vi "LS_DAQ_Cluster_RealTime.vi"() -> ()   [LabVIEW 2020]
uses:
  <vilib>/Platform/TimedLoop/XDataNode/timing_clust.ctl
  <vilib>/Platform/TimedLoop/XDataNode/nitl_modes.ctl
  <vilib>/Platform/TimedLoop/XDataNode/wakeup.ctl
  <vilib>/platform/TimedLoop/XDataNode/XDataNode.xnode
  <vilib>/Platform/TimedLoop/XDataNode/XDNodeRunTimeDep.lvlib
panel:
  out "Pulse count":dbl
  out "Period [ms]":u32
  out "Data":dbl[](array[numeric])
  out "error IO":errorcluster
  out "Finished Late? [i-1]":bool
  out "Iteration Duration":i64
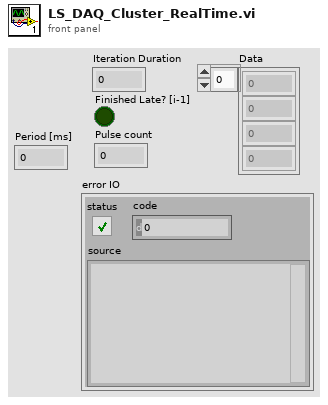
[diagram p1: front panel]
types:
  T1 = typedef "XDNodeRunTimeDep.lvlib/timing_clust.ctl" = cluster{"Expected End [f-1]":u64, "Actual End [f-1]":u64, "Finished Late? [f-1]":bool, "Expected End [i-1]":u64, "Actual End [i-1]":u64, "Finished Late? [i-1]":bool, "Expected Start [i]":u64, "Actual Start [i]":u64, "Expected Start [f]":u64, "Actual Start [f]":u64, "Source Name":string, "Structure Name":string, "Period":i64, "Deadline":i64, "Offset":i64, "Start":i64, "Priority":i32, "Timeout":i32, "Mode":T2, "Wakeup Reason":T3, "Error":errorcluster, "Source Type":string, "Secondary Source Type":string, "Global End Time":u64, "Global Start Time":u64, "Frame Duration":u64, "Iteration Duration":u64, "Assigned CPU":i32, "I/O Scan Engine Mode":u32}
  T2 = typedef "XDNodeRunTimeDep.lvlib/nitl_modes.ctl" = enum32{"No Change", "Process missed periods, maintain original phase", "Discard missed periods, maintain original phase", "Process missed periods, ignore original phase", "Discard missed periods, ignore original phase"}
  T3 = typedef "XDNodeRunTimeDep.lvlib/wakeup.ctl" = enum32{"Normal", "Aborted", "Asynchronous wakeup", "Timing source error", "Timed loop error", "Timeout"}
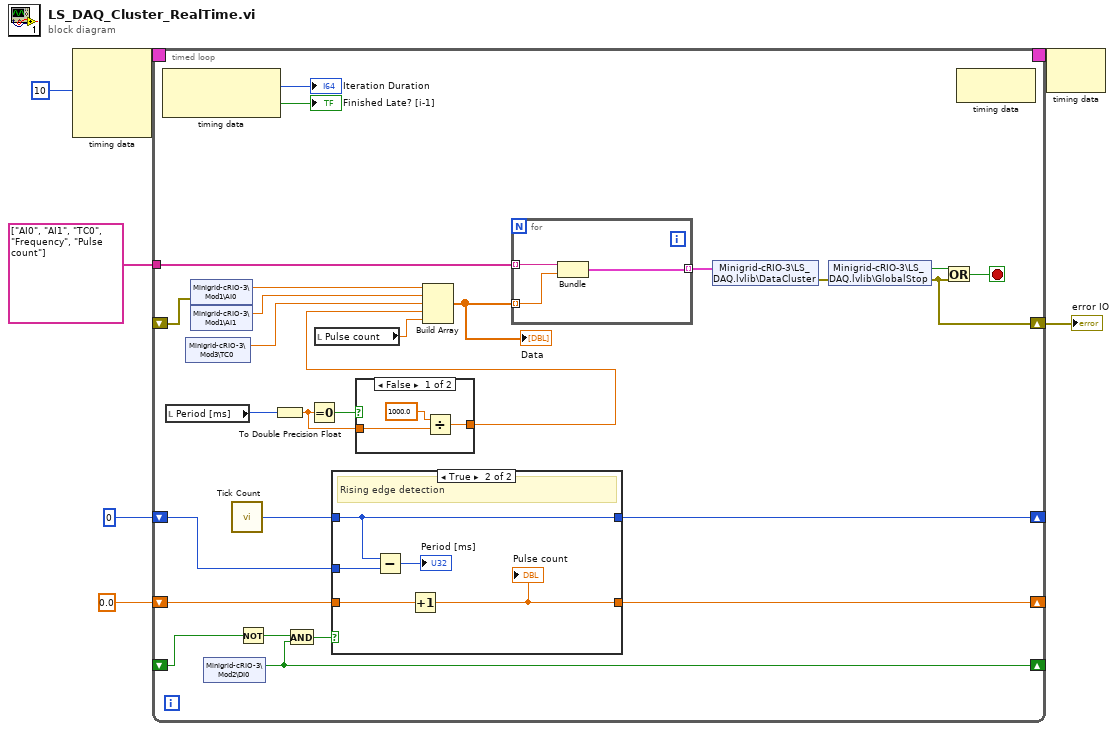
[diagram p0: block diagram]
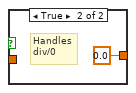
[diagram p2: hidden frame]
diagram:
  n1 = node-c288(i64 10 ("Period")) -> (w7:T1)  [unwired: 3 in]
  n2 = timed-loop {
    timing: w7 -> [_]
    timing-out: [_] -> w6
    shift-right: [w19] -> w2
    shift-left: _ -> [w31]
    shift-right: [w15] -> _
    shift-left: u32 0 ("Tick Count(uSec)") -> [w26]
    shift-right: [w25] -> _
    shift-left: _ -> [w24]
    shift-right: [w22] -> _
    shift-left: 0.0 ("Tick Count(uSec)") -> [w23]
    tunnel: string[] ["AI0", "AI1", "TC0", "Frequency", "Pulse count"] -> [w13]
    stop <- w21 stop-if-true
    n3 = node-c288() -> (→"Iteration Duration":i64, →"Finished Late? [i-1]":bool)  [unwired: 1 in]
    n4 = local read "Period [ms]"() -> (w18:u32)
    n5 = shared-variable "Minigrid-cRIO-3\\Mod3\\TC0"() -> (w8:dbl)  [unwired: 1 in, 1 out]
    n6 = shared-variable "Minigrid-cRIO-3\\Mod1\\AI0"(error in=w31) -> (w33:dbl, error out=w30:errorcluster)
    n7 = shared-variable "Minigrid-cRIO-3\\Mod1\\AI1"(error in=w30) -> (w32:dbl)  [unwired: 1 out]
    n8 = shared-variable "Minigrid-cRIO-3\\Mod2\\DI0"() -> (w25:bool)  [unwired: 1 in, 1 out]
    n9 = call "Tick Count"() -> ("Tick Count(mSec)"=w27:u32)
    n10 = Not(x=w24) -> (.not. x?=w29:bool)
    n11 = To Double Precision Float(number=w18) -> (double precision float=w16:dbl)
    n12 = And(x=w29, y=w25) -> (x .and. y?=w28:bool)
    n13 = Equal To 0?(x=w16) -> (x = 0?=w17:bool)
    n14 = local read "Pulse count"() -> (w10:dbl)
    n15 = case shown="True" w28 {
      tunnel: w27 -> [_ w45]
      tunnel: w26 -> [w43 w49]
      tunnel: w23 -> [w44 w47]
      tunnel: [w44 w46] -> w22
      tunnel: [w43 w45] -> w15
      frame False {
      }
      frame True {
        # "Rising edge detection"
        n16 = Subtract(x=w45, y=w49) -> (x-y=→"Period [ms]":u32)
        n17 = Increment(x=w47) -> (x+1=w46:dbl)
        "Pulse count" <- w46
      }
    }
    n18 = case shown="False" w17 {
      tunnel: w16 -> [w41 _]
      tunnel: [w39 0.0] -> w9
      frame False {
        n19 = Divide(x=1000.0, y=w41) -> (x/y=w39:dbl)
      }
      frame True {
        # "Handles\ndiv/0"
      }
    }
    n20 = Build Array(w33, w32, w8, w9, w10) -> (w14:dbl[])
    "Data" <- w14
    n21 = for {
      tunnel: w14 -> [w37] mode=indexing
      tunnel: w13 -> [w38] mode=indexing
      tunnel: [w36] -> w12 mode=indexing
      n22 = Bundle(w38, "Pulse count"=w37) -> (w36:cluster{string, "Pulse count":dbl})  [unwired: 1 in]
    }
    n23 = shared-variable "Minigrid-cRIO-3\\LS_DAQ.lvlib\\DataCluster"(w12) -> (error out=w11:errorcluster)  [unwired: 1 in]
    n24 = shared-variable "Minigrid-cRIO-3\\LS_DAQ.lvlib\\GlobalStop"(error in=w11) -> (w20:bool, error out=w19:errorcluster)
    n25 = Or(x=w20, y=w19) -> (x .or. y?=w21:bool)
    n26 = node-c288() -> ()  [unwired: 1 in, 1 out]
  }
  "error IO" <- w2
  n27 = node-c288(w6) -> ()  [unwired: 1 out]
